vi "Read Amount.vi"(8 "error in (no error)":errorcluster, 11 "AReceipt in":refnum<class "AReceipt.lvclass">) -> (0 "error out":errorcluster, 2 "Amount":dbl, 3 "AReceipt out":refnum<class "AReceipt.lvclass">)   [LabVIEW 2020, in "AReceipt.lvclass"]
uses:
  AReceipt.lvclass
  AReceipt.lvclass/AReceipt.ctl
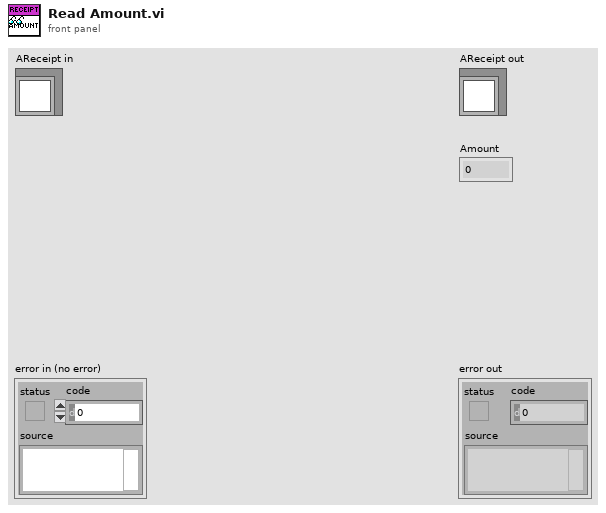
[diagram p1: front panel]
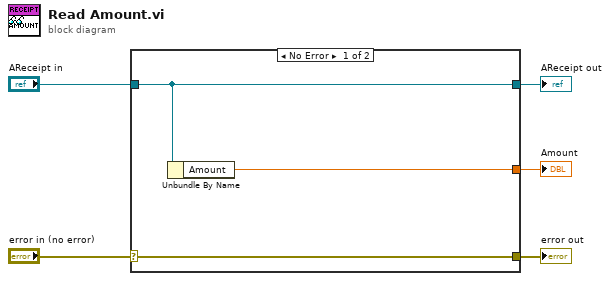
[diagram p0: block diagram]
diagram:
  n1 = case shown="No Error" "error in (no error)" {
    selector: "error in (no error)" -> [w8 w9]
    tunnel: [w8 w9] -> w4
    tunnel: [w7 w10] -> w2
    tunnel: "AReceipt in" -> [w7 w10]
    tunnel: [w6 _] -> w1
    frame No Error {
      n2 = Unbundle By Name(w7) -> ("Amount"=w6:dbl)
    }
    frame Error {
    }
  }
  "error out" <- w4
  "AReceipt out" <- w2
  "Amount" <- w1
